vi "Multiple Reads.vi"() -> ()   [LabVIEW 2021]
uses:
  <vilib>/Analysis/2dsp.llb/Complex FFT.vi
  VIs/Initialize by Serial.vi
  RTL-SDR.lvlib
  <vilib>/Analysis/NI_AALPro.lvlib
panel:
  out "FFT Graph 2":cluster{"f0":dbl, "df":dbl, "Y":dbl[]}(graph)
  in  "# Reads":i32=100
  out "error out":errorcluster
  in  "FFT size":i32=8192
  out "FFT Graph":cluster{"f0":dbl, "df":dbl, "Y":dbl[]}[](graph)
  out "Actual Sample Rate (Hz)":u32 format="%#.6p"
  in  "Sample Rate (Hz)":u32=2000000 format="%#.6p"
  out "Manufacturer Name":string
  out "Product Name":string
  out "Serial Number":string
  in  "Center Frequency (Hz)":u32=80000000 format="%#_6p"
  out "Actual Center Frequency (Hz)":u32 format="%#.6p"
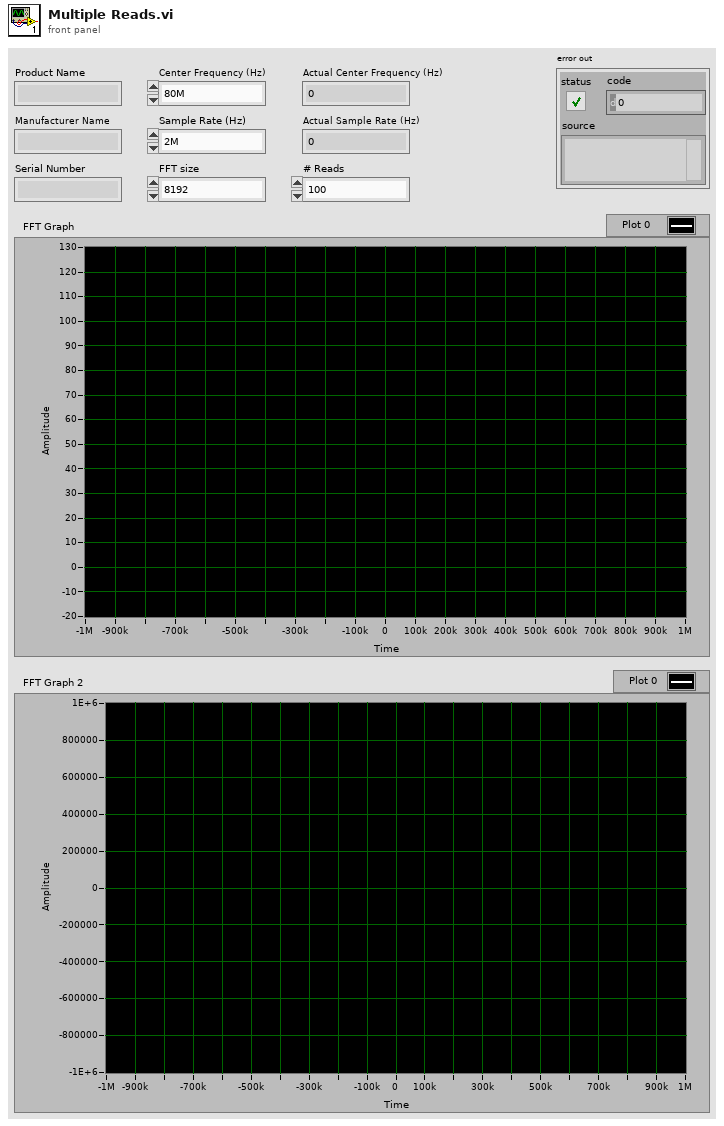
[diagram p1: front panel]
types:
  T1 = typedef "RTL-SDR.lvlib/Device Handle.ctl" = u64
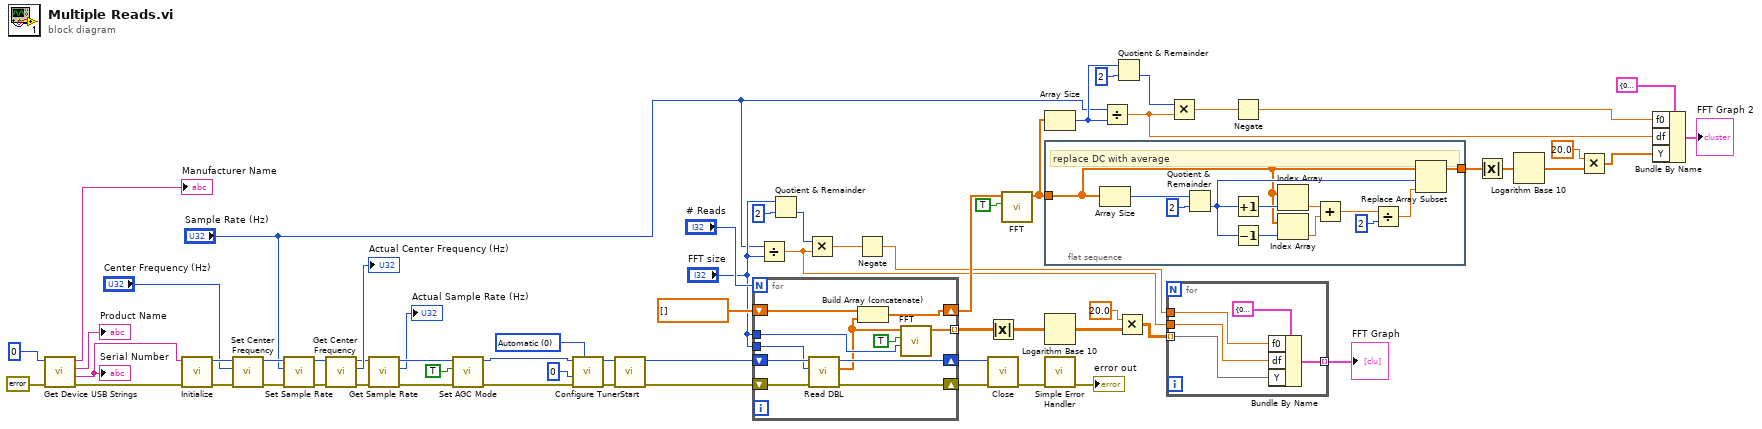
[diagram p0: block diagram]
diagram:
  w44 = u16 0 items=["Automatic", "Manual"] ("Tuner Gain Mode")
  n1 = call "Get Device USB Strings.vi"("error in (no error)"=errorcluster {"status"=FALSE, "code"=0, "source"=""} ("error in"), "device index"=u32 0) -> ("error out"=w62:errorcluster, "Serial Number"=w58:string, "Product Name"=→"Product Name":string, "Manufacturer Name"=→"Manufacturer Name":string)  [unwired: 6 in]
  "Serial Number" <- w58
  n2 = call-poly "Initialize.vi"("error in (no error)"=w62, "Serial Number"=w58) -> ("error out"=w55:errorcluster, "device handle out"=w56:T1)  [unwired: 8 in]
  n3 = call "Set Center Frequency.vi"("error in (no error)"=w55, "Center Frequency (Hz)"="Center Frequency (Hz)", "device handle in"=w56) -> ("error out"=w29:errorcluster, "device handle out"=w30:T1)  [unwired: 7 in]
  n4 = call "Set Sample Rate.vi"("error in (no error)"=w29, "Sample Rate (Hz)"="Sample Rate (Hz)", "device handle in"=w30) -> ("error out"=w51:errorcluster, "device handle out"=w50:T1)  [unwired: 7 in]
  n5 = call "Get Center Frequency.vi"("error in (no error)"=w51, "device handle in"=w50) -> ("error out"=w31:errorcluster, "Center Frequency (Hz)"=→"Actual Center Frequency (Hz)":u32, "device handle out"=w32:T1)  [unwired: 7 in]
  n6 = call "Get Sample Rate.vi"("error in (no error)"=w31, "device handle in"=w32) -> ("error out"=w41:errorcluster, "Sample Rate (Hz)"=→"Actual Sample Rate (Hz)":u32, "device handle out"=w42:T1)  [unwired: 7 in]
  n7 = call "Set AGC Mode.vi"("error in (no error)"=w41, "Enable AGC (T)"=TRUE, "device handle in"=w42) -> ("error out"=w47:errorcluster, "device handle out"=w46:T1)  [unwired: 7 in]
  n8 = call "Configure Tuner.vi"("Tuner Gain Mode (0: auto)"=w44, "error in (no error)"=w47, "Bandwidth (Hz) (0: auto)"=u32 0, "device handle in"=w46) -> ("error out"=w40:errorcluster, "device handle out"=w27:T1)  [unwired: 6 in]
  n9 = call "Start.vi"("error in (no error)"=w40, "device handle in"=w27) -> ("error out"=w52:errorcluster, "device handle out"=w26:T1)  [unwired: 8 in]
  n10 = for {
    N: "# Reads" -> [_]
    tunnel: "FFT size" -> [w70]
    shift-right: [w74] -> w57
    shift-left: w52 -> [w73]
    shift-right: [w72] -> w28
    shift-left: w26 -> [w71]
    tunnel: "FFT size" -> [w69]
    tunnel: [w67] -> w24 mode=indexing
    shift-right: [w64] -> w20
    shift-left: cdb[] [] -> [w65]
    n11 = call "Read DBL.vi"("error in (no error)"=w73, "# samples"=w70, "device handle in"=w71) -> ("error out"=w74:errorcluster, "Data"=w66:cdb[], "device handle out"=w72:T1)  [unwired: 6 in]
    n12 = Build Array (concatenate)(w65, w66) -> (w64:cdb[])
    n13 = call-poly <vilib>:"FFT.vi"("FFT size"=w69, "shift?"=TRUE, "X"=w66) -> ("FFT {X}"=w67:cdb[])  [unwired: 7 in, 1 out]
  }
  n14 = Divide(x="Sample Rate (Hz)", y="FFT size") -> (x/y=w16:dbl)
  n15 = Quotient & Remainder(x="FFT size", y=2) -> (floor(x/y)=w33:i32)  [unwired: 1 out]
  n16 = Multiply(x=w33, y=w16) -> (x*y=w34:dbl)
  n17 = Negate(x=w34) -> (-x=w9:dbl)
  n18 = Absolute Value(x=w24) -> (abs(x)=w36:dbl[][])
  n19 = call "Close.vi"("error in"=w57, "device handle in"=w28) -> ("error out"=w54:errorcluster)  [unwired: 9 in]
  n20 = call-poly <vilib>:"FFT.vi"("shift?"=TRUE, "X"=w20) -> ("FFT {X}"=w6:cdb[])  [unwired: 8 in, 1 out]
  n21 = Array Size(array=w6) -> (size(s)=w11:i32)
  n22 = flat-sequence {
    tunnel: w6 -> [w79]
    tunnel: [w75] -> w2
    frame #0 {
      # "replace DC with average"
      n23 = Array Size(array=w79) -> (size(s)=w86:i32)
      n24 = Quotient & Remainder(x=w86, y=2) -> (floor(x/y)=w82:i32)  [unwired: 1 out]
      n25 = Increment(x=w82) -> (x+1=w83:i32)
      n26 = Decrement(x=w82) -> (x-1=w84:i32)
      n27 = Index Array(array=w79, index=w83) -> (element=w81:cdb)
      n28 = Index Array(array=w79, index=w84) -> (element=w80:cdb)
      n29 = Add(x=w81, y=w80) -> (x+y=w78:cdb)
      n30 = Divide(x=w78, y=2) -> (x/y=w76:cdb)
      n31 = Replace Array Subset(array=w79, new element=w76, index=w82) -> (w75:cdb[])
    }
  }
  n32 = Logarithm Base 10(1:w36) -> (0:w38:dbl[][])
  n33 = call <vilib>:"Simple Error Handler.vi"("error in (no error)"=w54) -> ("error out"=→"error out":errorcluster)  [unwired: 4 in, 4 out]
  n34 = Divide(x="Sample Rate (Hz)", y=w11) -> (x/y=w7:dbl)
  n35 = Quotient & Remainder(x=w11, y=2) -> (floor(x/y)=w12:i32)  [unwired: 1 out]
  n36 = Multiply(x=20.0, y=w38) -> (x*y=w22:dbl[][])
  n37 = for {
    tunnel: w9 -> [w91]
    tunnel: w16 -> [w90]
    tunnel: [w88] -> w23 mode=indexing
    tunnel: w22 -> [w87] mode=indexing
    n38 = Bundle By Name(cluster=cluster{"f0":dbl, "df":dbl, "Y":dbl[]} {"f0"=0.0, "df"=0.0, "Y"=[]}, "f0"=w91, "df"=w90, "Y"=w87) -> (w88:cluster{"f0":dbl, "df":dbl, "Y":dbl[]})
  }
  "FFT Graph" <- w23
  n39 = Multiply(x=w12, y=w7) -> (x*y=w13:dbl)
  n40 = Negate(x=w13) -> (-x=w8:dbl)
  n41 = Absolute Value(x=w2) -> (abs(x)=w3:dbl[])
  n42 = Logarithm Base 10(1:w3) -> (0:w5:dbl[])
  n43 = Multiply(x=20.0, y=w5) -> (x*y=w1:dbl[])
  n44 = Bundle By Name(cluster=cluster{"f0":dbl, "df":dbl, "Y":dbl[]} {"f0"=0.0, "df"=0.0, "Y"=[]}, "f0"=w8, "df"=w7, "Y"=w1) -> (→"FFT Graph 2":cluster{"f0":dbl, "df":dbl, "Y":dbl[]})
